vi "Main.vi"(8 "error in (no error)":errorcluster, 11 "Process in":refnum<class "Sine Process.lvclass">) -> (0 "error out":errorcluster, 3 "Process out":refnum<class "Sine Process.lvclass">)   [LabVIEW 2019, in "TimingDRV Engine.lvlib" / "Sine Process.lvclass"]
uses:
  Sine Process.lvclass
  C:/Users/XEnderMD/Desktop/CD Project Tools/Source/Engine/Parent Classes/Process/Process.lvclass
  Parent Classes/Process/Process.lvclass/Process.ctl
  <vilib>/Platform/TimedLoop/XDataNode/timing_clust.ctl
  <vilib>/Platform/TimedLoop/XDataNode/nitl_modes.ctl
  <vilib>/Platform/TimedLoop/XDataNode/wakeup.ctl
  <vilib>/platform/TimedLoop/XDataNode/XDataNode.xnode
  Parent Classes/Process/Process.lvclass
  <vilib>/Platform/TimedLoop/XDataNode/XDNodeRunTimeDep.lvlib
  <vilib>/NI VeriStand/Custom Device API/Custom Device API.lvlib
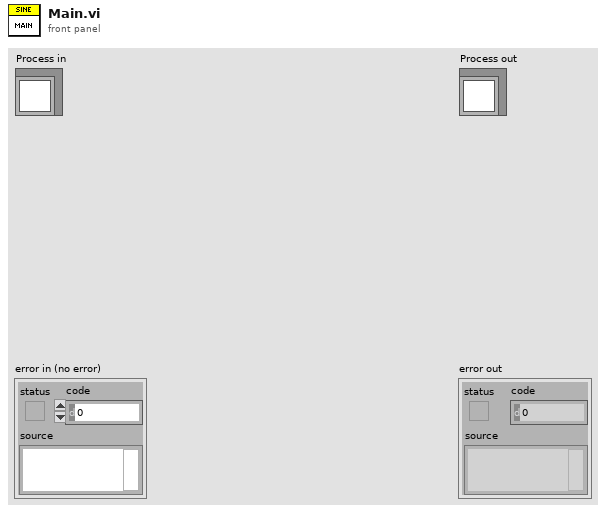
[diagram p1: front panel]
types:
  T1 = typedef "XDNodeRunTimeDep.lvlib/timing_clust.ctl" = cluster{"Expected End [f-1]":u64, "Actual End [f-1]":u64, "Finished Late? [f-1]":bool, "Expected End [i-1]":u64, "Actual End [i-1]":u64, "Finished Late? [i-1]":bool, "Expected Start [i]":u64, "Actual Start [i]":u64, "Expected Start [f]":u64, "Actual Start [f]":u64, "Source Name":string, "Structure Name":string, "Period":i64, "Deadline":i64, "Offset":i64, "Start":i64, "Priority":i32, "Timeout":i32, "Mode":T2, "Wakeup Reason":T3, "Error":errorcluster, "Source Type":string, "Secondary Source Type":string, "Global End Time":u64, "Global Start Time":u64, "Frame Duration":u64, "Iteration Duration":u64, "Assigned CPU":i32, "I/O Scan Engine Mode":u32}
  T2 = typedef "XDNodeRunTimeDep.lvlib/nitl_modes.ctl" = enum32{"No Change", "Process missed periods, maintain original phase", "Discard missed periods, maintain original phase", "Process missed periods, ignore original phase", "Discard missed periods, ignore original phase"}
  T3 = typedef "XDNodeRunTimeDep.lvlib/wakeup.ctl" = enum32{"Normal", "Aborted", "Asynchronous wakeup", "Timing source error", "Timed loop error", "Timeout"}
  T4 = typedef "TimingDRV Engine.lvlib/Process.lvclass/Async Paramters.ctl" = cluster{"Device Reference":T5, "Device Clock":string, "Device Inputs FIFO":refnum<k33>, "Device Outputs FIFO":refnum<k33>, "CD Engine Event Ref":T6}
  T5 = typedef "Custom Device API.lvlib/Custom Device Item Ref.ctl" = u64
  T6 = typedef "Custom Device API.lvlib/Custom Device Engine Event Ref.ctl" = refnum<event-registration>
  T7 = typedef "Custom Device API.lvlib/Custom Device Timed Loop Priority.ctl" = enum32{"Low", "Medium", "High"}
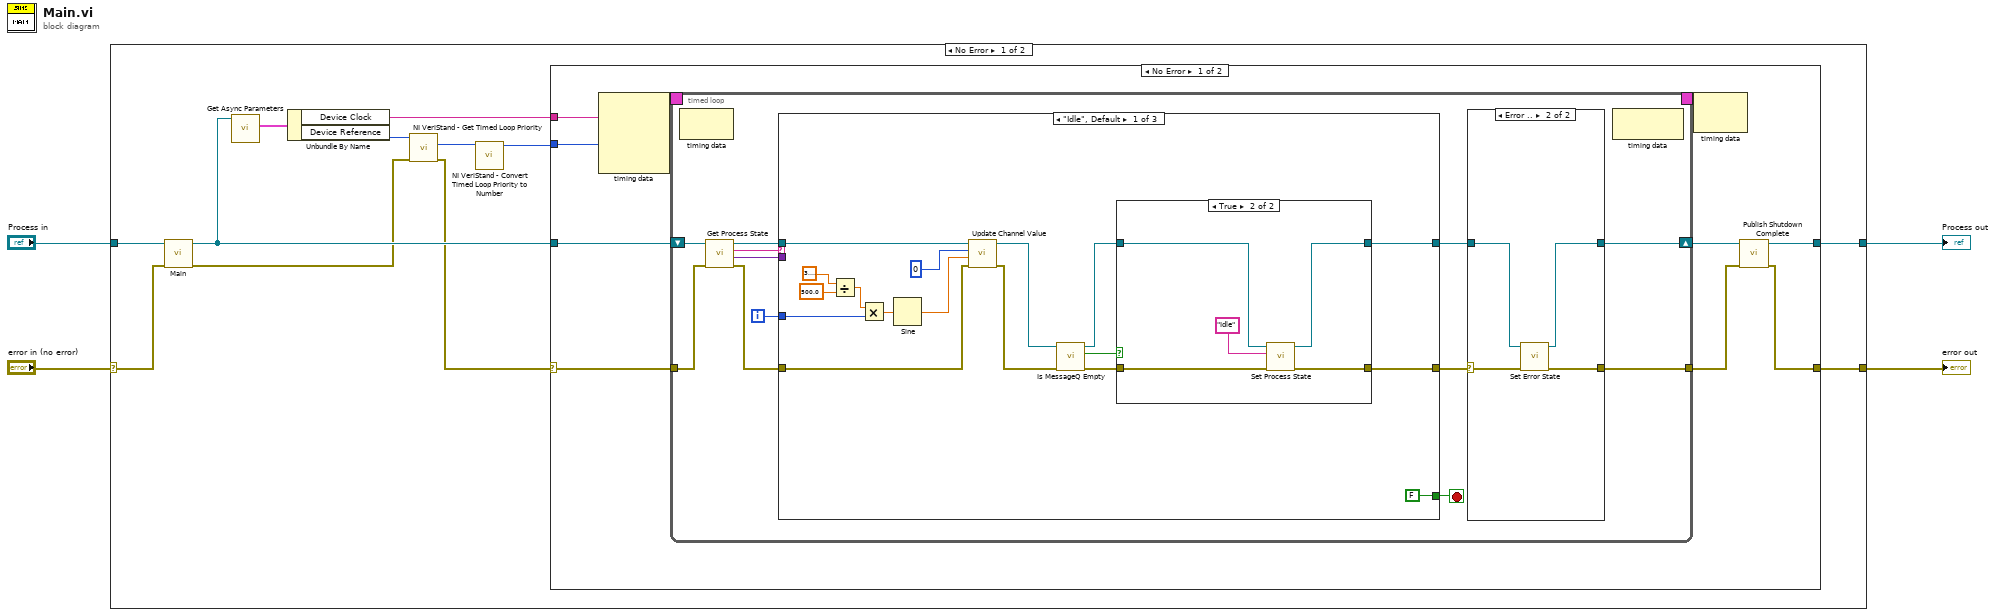
[diagram p0: block diagram]
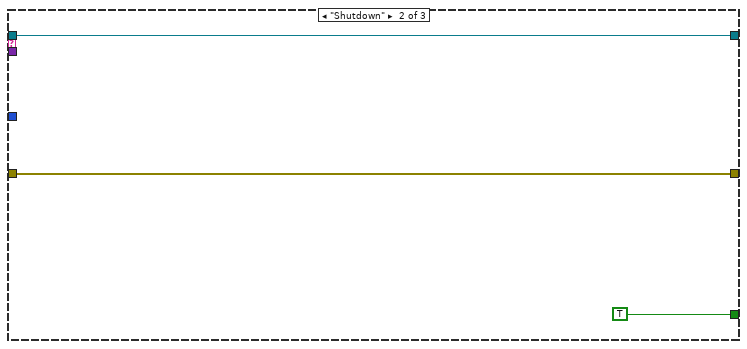
[diagram p4: hidden frame]
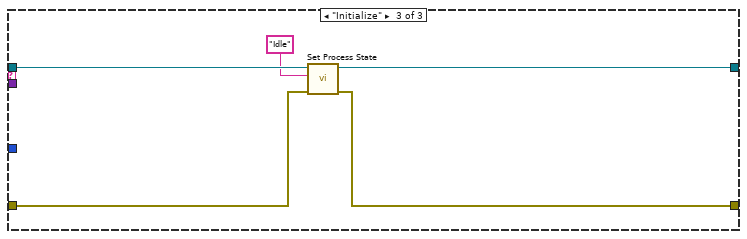
[diagram p5: hidden frame]
diagram:
  n1 = case shown="No Error" "error in (no error)" {
    selector: "error in (no error)" -> [w15 w87]
    tunnel: [w13 w87] -> w1
    tunnel: [w14 w86] -> w2
    tunnel: "Process in" -> [w16 w86]
    frame No Error {
      n2 = call-parent "Main.vi"("error in (no error)"=w15, "Process in"=w16) -> ("error out"=w8:errorcluster, "Process out"=w12:refnum<class "Sine Process.lvclass">)  [unwired: 8 in]
      n3 = call "Get Async Parameters.vi"("Process in"=w12) -> ("Async Parameters"=w11:T4)  [unwired: 9 in, 1 out]
      n4 = Unbundle By Name(w11) -> ("Device Clock"=w10:string, "Device Reference"=w9:T5)
      n5 = call <vilib>:"NI VeriStand - Get Timed Loop Priority.vi"("error in (no error)"=w8, "Device Ref in"=w9) -> ("error out"=w5:errorcluster, "Priority"=w7:T7)  [unwired: 7 in, 1 out]
      n6 = call <vilib>:"NI VeriStand - Convert Timed Loop Priority to Number.vi"("Priority"=w7) -> ("Numeric Priority"=w6:i32)  [unwired: 10 in]
      n7 = case shown="No Error" w5 {
        selector: w5 -> [w17 w84]
        tunnel: [w23 w85] -> w14
        tunnel: [w21 w84] -> w13
        tunnel: w12 -> [w20 w85]
        tunnel: w10 -> [w19 _]
        tunnel: w6 -> [w18 _]
        frame No Error {
          n8 = node-c288(w19, w18) -> (w26:T1)  [unwired: 2 in]
          n9 = timed-loop {
            shift-right: [w31] -> w24
            shift-left: w20 -> [w37]
            tunnel: w17 -> [w38]
            tunnel: [w30] -> w22
            timing: w26 -> [_]
            timing-out: [_] -> w25
            i -> [w27]
            stop <- w29 stop-if-true
            n10 = node-c288() -> ()  [unwired: 1 in, 1 out]
            n11 = call "Get Process State.vi"("error in (no error)"=w38, "Process in"=w37) -> ("error out"=w34:errorcluster, "Payload"=w35:variant, "Command"=w28:string, "Process out"=w36:refnum<class "Sine Process.lvclass">)  [unwired: 6 in]
            n12 = case shown="\"Idle\", Default" w28 {
              tunnel: w36 -> [w62 w73 w78]
              tunnel: w35 -> [_ _ _]
              tunnel: w34 -> [w61 w72 w77]
              tunnel: [w54 w73 w76] -> w33
              tunnel: [w53 w72 w75] -> w32
              tunnel: [FALSE TRUE _] -> w29
              tunnel: w27 -> [w50 _ _]
              frame "Idle", Default {
                n13 = Divide(x=3.141592653589793, y=500.0) -> (x/y=w49:dbl)
                n14 = Multiply(x=w49, y=w50) -> (x*y=w48:dbl)
                n15 = Sine(x=w48) -> (sin(x)=w47:dbl)
                n16 = call "Update Channel Value.vi"("error in (no error)"=w61, "New Value"=w47, "Channel Index"=0, "Output Process in"=w62) -> ("error out"=w59:errorcluster, "Output Process out"=w58:refnum<class "Sine Process.lvclass">)  [unwired: 4 in, 2 out]
                n17 = call "Is MessageQ Empty.vi"("error in (no error)"=w59, "Process in"=w58) -> ("error out"=w56:errorcluster, "is Empty ?"=w57:bool, "Process out"=w55:refnum<class "Sine Process.lvclass">)  [unwired: 7 in]
                n18 = case shown="True" w57 {
                  tunnel: w56 -> [w64 w66]
                  tunnel: w55 -> [w65 w69]
                  tunnel: [w65 w68] -> w54
                  tunnel: [w64 w67] -> w53
                  frame False {
                  }
                  frame True {
                    n19 = call "Set Process State.vi"("error in (no error)"=w66, "Command"="Idle", "Process in"=w69) -> ("error out"=w67:errorcluster, "Process out"=w68:refnum<class "Sine Process.lvclass">)  [unwired: 7 in]
                  }
                }
              }
              frame "Shutdown" {
              }
              frame "Initialize" {
                n20 = call "Set Process State.vi"("error in (no error)"=w77, "Command"="Idle", "Process in"=w78) -> ("error out"=w75:errorcluster, "Process out"=w76:refnum<class "Sine Process.lvclass">)  [unwired: 7 in]
              }
            }
            n21 = case shown="Error .." w32 {
              selector: w32 -> [w41 w46]
              tunnel: w33 -> [w42 w45]
              tunnel: [w42 w44] -> w31
              tunnel: [w41 w43] -> w30
              frame No Error {
              }
              frame Error {
                n22 = call "Set Error State.vi"("error in (no error)"=w46, "Process in"=w45) -> ("error out"=w43:errorcluster, "Process out"=w44:refnum<class "Sine Process.lvclass">)  [unwired: 8 in]
              }
            }
            n23 = node-c288() -> ()  [unwired: 1 in, 1 out]
          }
          n24 = node-c288(w25) -> ()  [unwired: 1 out]
          n25 = call "Publish Shutdown Complete.vi"("error in (no error)"=w22, "Process in"=w24) -> ("error out"=w21:errorcluster, "Process out"=w23:refnum<class "Sine Process.lvclass">)  [unwired: 8 in]
        }
        frame Error {
        }
      }
    }
    frame Error {
    }
  }
  "error out" <- w1
  "Process out" <- w2
